vi "Stop.vi"   [LabVIEW 2014]
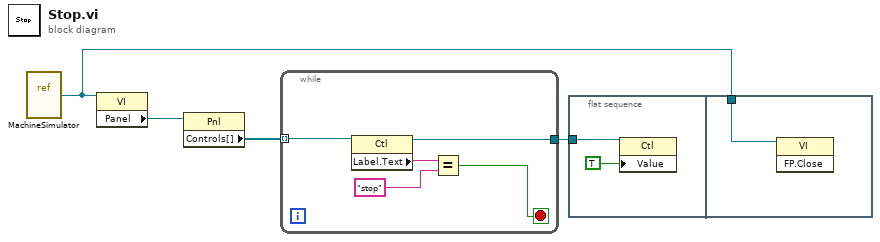
[diagram p0: block diagram]
diagram:
  n1 = vi-ref "MachineSimulator.vi"() -> (w1:refnum<vi>)
  n2 = property class="VI"(reference=w1) -> ("Panel"=w2:refnum<vi>)  [unwired: 1 in, 2 out]
  n3 = property class="Pnl"(reference=w2) -> ("Controls[]"=w4:refnum<vi>[])  [unwired: 1 in, 2 out]
  n4 = while {
    tunnel: w4 -> [w9] mode=indexing
    tunnel: [w5] -> w3
    stop <- w6 stop-if-true
    n5 = property class="Ctl"(reference=w9) -> (reference out=w5:refnum<vi>, "Label.Text"=w8:string)  [unwired: 1 in, 1 out]
    n6 = Equal?(x=w8, y="stop") -> (x = y?=w6:bool)
  }
  n7 = flat-sequence {
    tunnel: w3 -> [w11]
    tunnel: w1 -> [w12]
    frame #0 {
      n8 = property class="Ctl"(reference=w11, "Value"=TRUE) -> ()  [unwired: 1 in, 2 out]
    }
    frame #1 {
      n9 = invoke class="VI" method="FP.Close"(reference=w12) -> ()  [unwired: 2 in, 3 out]
    }
  }
